vi "Test Drift.vi"() -> ()   [LabVIEW 2020]
uses:
  Labview Library/Libraries/Basic Experiment/Basic Experiment.lvlib
panel:
  in  "stop":bool
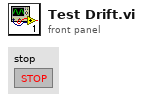
[diagram p1: front panel]
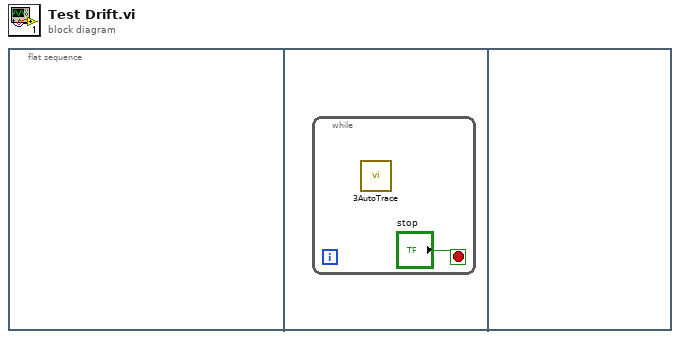
[diagram p0: block diagram]
diagram:
  n1 = flat-sequence {
    frame #0 {
    }
    frame #1 {
      n2 = while {
        stop <- "stop" stop-if-true
        n3 = call "3AutoTrace.vi"() -> ()  [unwired: 7 in, 3 out]
      }
    }
    frame #2 {
    }
  }
